vi "RS64_ext.vi"(3 "Q old":u64 format="%x", 4 "R":u64 format="%x", 5 "S":u64 format="%x") -> (1 "~Q":u64=4294967295 format="%x", 2 "Q":u64 format="%x")   [LabVIEW 2019, in "Triggers.lvlib"]
uses:
  Triggers.lvlib
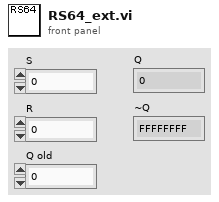
[diagram p1: front panel]
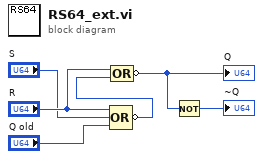
[diagram p0: block diagram]
diagram:
  n1 = Compound Arithmetic op=OR("R", "S", "Q old") -> (invert w5:u64)
  n2 = Compound Arithmetic op=OR("R", w5) -> (invert w3:u64)
  "Q" <- w3
  n3 = Not(x=w3) -> (.not. x?=→"~Q":u64)
